vi "MPU panel.vi"() -> (0 "Error Out":errorcluster, 3 "VISA resource out":refnum<visa-resource-name>)   [LabVIEW 2016]
uses:
  <vilib>/Math Plots/3D Math Plots/3D Scatter/3D Scatter XCtrl/3D Scatter.xctl
  <vilib>/BLE/type_def/connection_status_bundle.ctl
  <vilib>/BLE/type_def/address_type.ctl
  Typedef/MPU panel - States.ctl
  Typedef/BLE char handle.ctl
  <vilib>/Math Plots/3D Math Plots/3D Scatter/3D Scatter Datatype/Public/Plot Helper (Vector).vi
  <vilib>/Math Plots/3D Math Plots/3D Scatter/3D Scatter Datatype/3D Scatter Datatype.lvclass
panel:
  in  "VISA resource in":refnum<visa-resource-name>
  in  "Calib Gyro":bool
  in  "Calib Mag":bool
  in  "Calib Accel":bool
  out "GyroZ":dbl caption="Z" format="%#_gdps"
  out "GyroY":dbl caption="Y" format="%#_gdps"
  out "GyroX":dbl caption="X" format="%#_gdps"
  out "Gyroscope Chart":cluster{"[0]":dbl, "[1]":dbl, "[2]":dbl}(graph)
  out "AccZ":dbl caption="Z" format="%#_gg"
  out "AccY":dbl caption="Y" format="%#_gg"
  out "AccX":dbl caption="X" format="%#_gg"
  out "Accelerometer Chart":cluster{"[0]":dbl, "[1]":dbl, "[2]":dbl}(graph)
  in  "Connection Status":T1={"MAC Address"="", "cnx handle"=0, "cnx flags"=0, "Address Type"=125, "Connection Interval (ms)"=125, "Timeout(ms)"=125, "Latency"=0, "bonding handle"=0} {"Address Type" items=["Public", "Random"]}
  in  "Clear Plot":bool
  out "3D Mag Scatter":refnum<class "3D Plot Datatype.lvclass">[](xcontrol)
  in  "Acquire MPU":bool
  # "Points [N]"
  # "Points [N]"
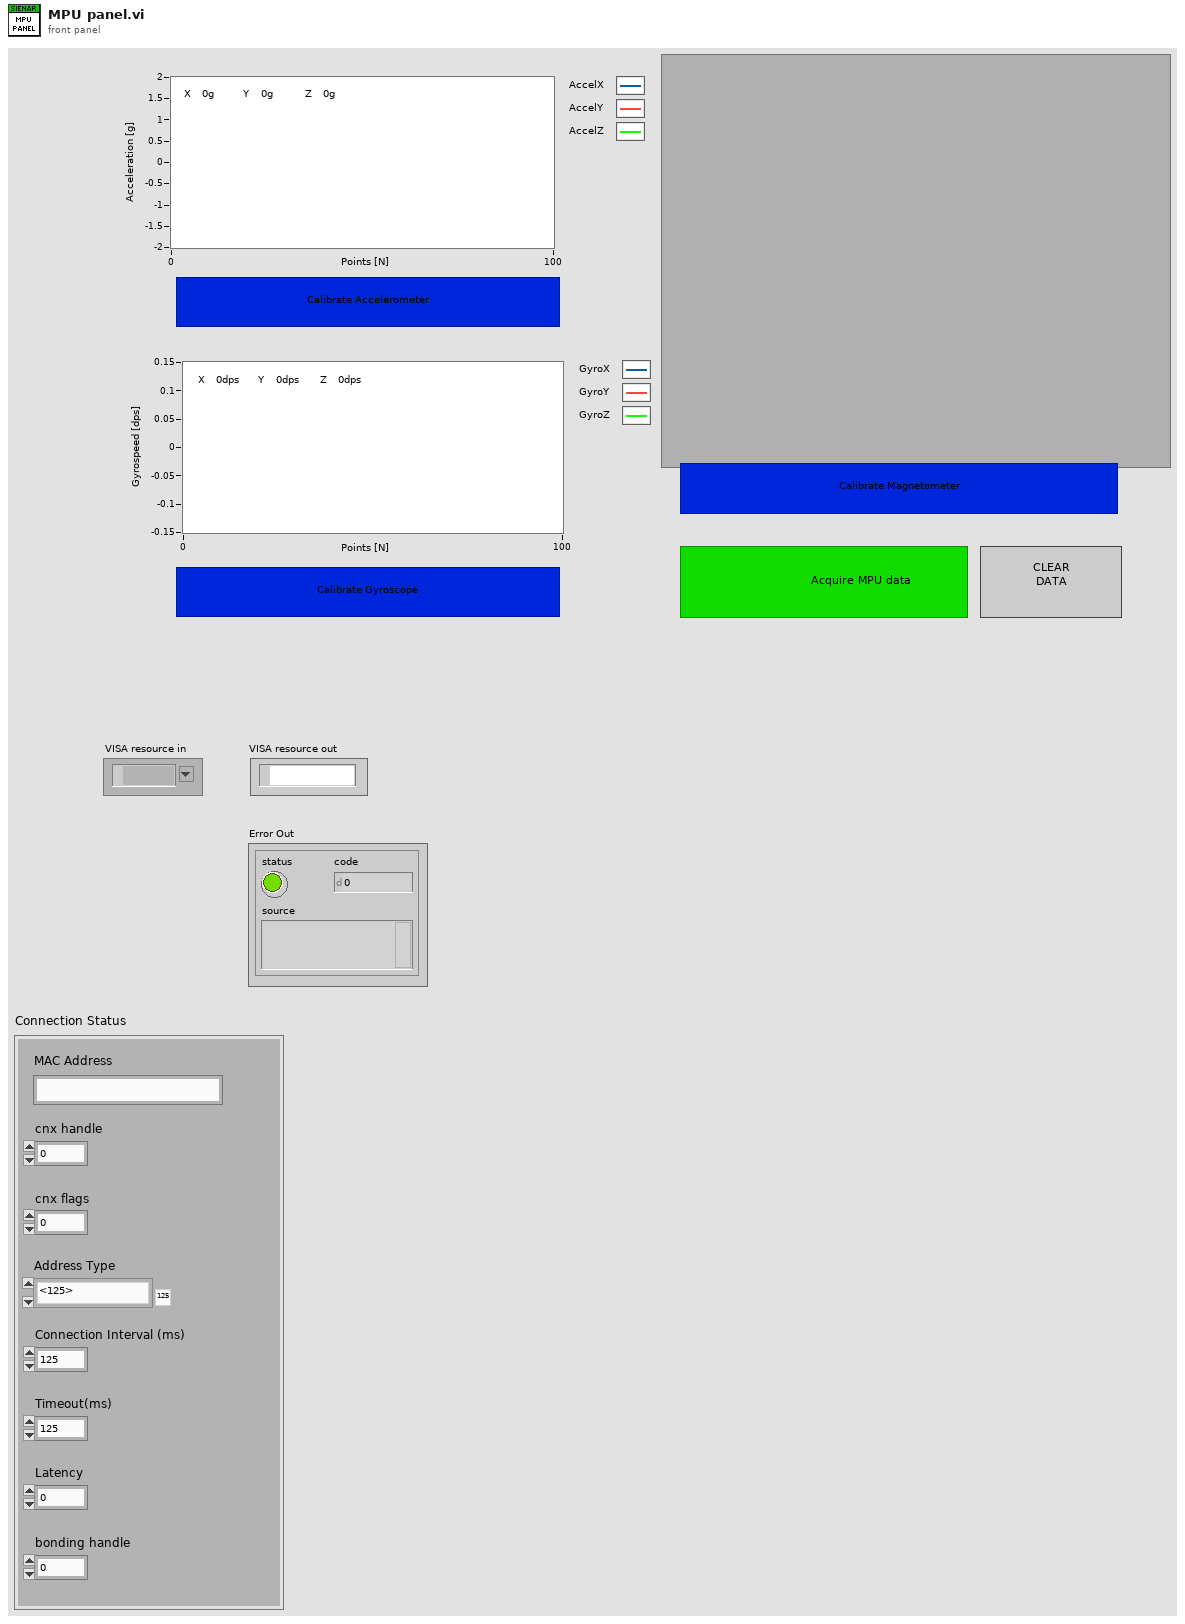
[diagram p1: front panel]
types:
  T1 = typedef "connection_status_bundle.ctl" = cluster{"MAC Address":string, "cnx handle":u8, "cnx flags":u8, "Address Type":T2, "Connection Interval (ms)":u16, "Timeout(ms)":u16, "Latency":u16, "bonding handle":u8}
  T2 = typedef "address_type.ctl" = u8
  T3 = typedef "MPU panel - States.ctl" = enum16{"Read MPU data", "Stop", "Calib Accelerometer", "Calib Gyroscope", "Calib Magnetometer", "Clear Plots", "Exit"}
  T4 = typedef "BLE char handle.ctl" = u16
  T5 = cluster{"AccelData":cluster{"AccelX":i16, "AccelY":i16, "AccelZ":i16}, "GyroData":cluster{"GyroX":i16, "GyroY":i16, "GyroZ":i16}, "MagData":cluster{"MagX":i16, "MagY":i16, "MagZ":i16}}
  T6 = cluster{"AccelData":cluster{"AccelX":dbl, "AccelY":dbl, "AccelZ":dbl}, "GyroData":cluster{"GyroX":dbl, "GyroY":dbl, "GyroZ":dbl}, "MagData":cluster{"MagX":dbl, "MagY":dbl, "MagZ":dbl}}
  T7 = cluster{"AccelX":dbl, "AccelY":dbl, "AccelZ":dbl}
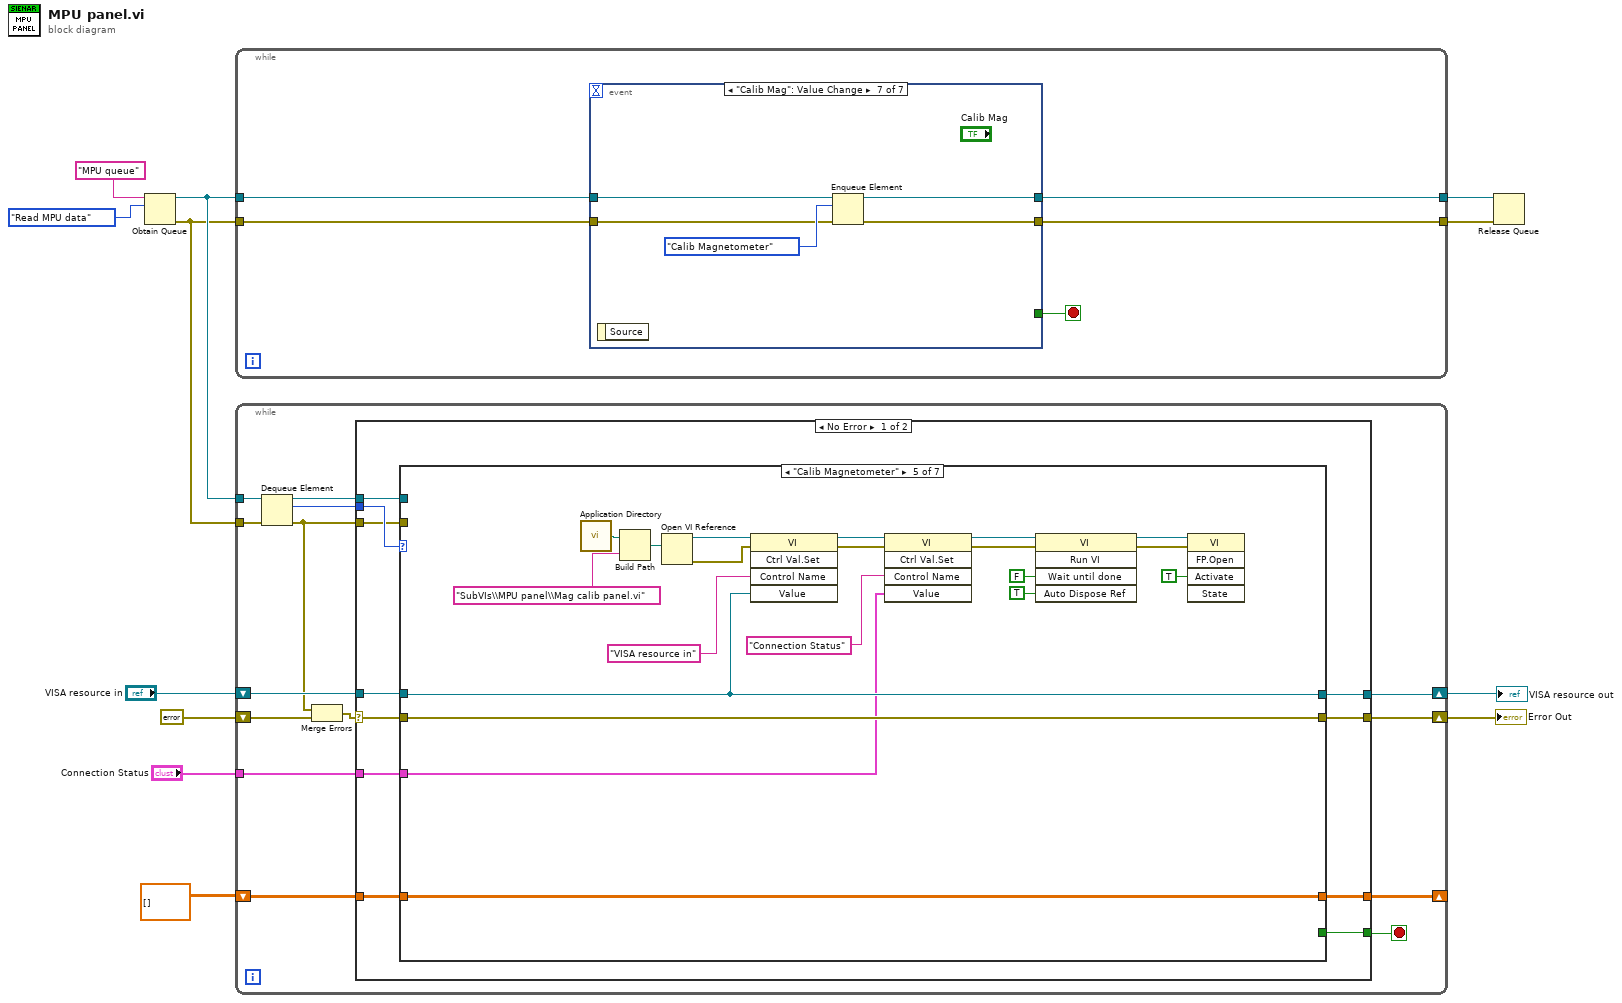
[diagram p0: block diagram]
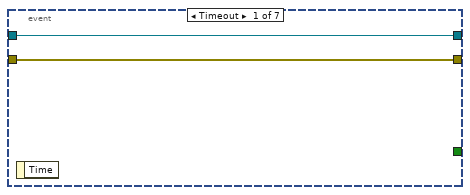
[diagram p2: hidden frame]
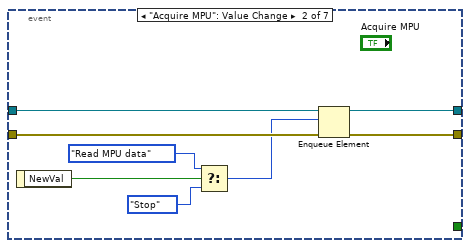
[diagram p3: hidden frame]
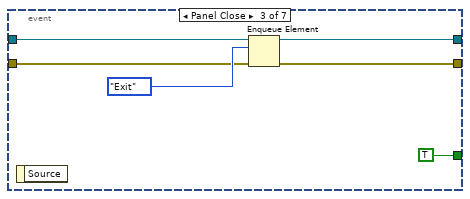
[diagram p4: hidden frame]
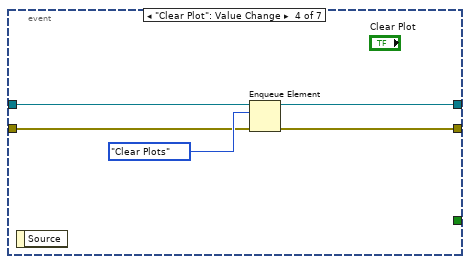
[diagram p5: hidden frame]
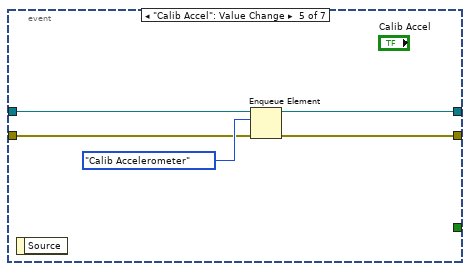
[diagram p6: hidden frame]
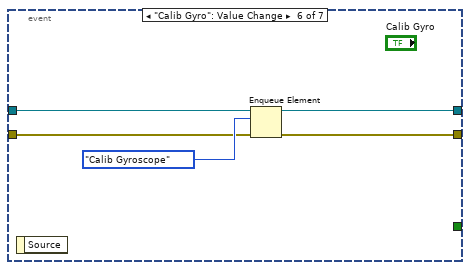
[diagram p7: hidden frame]
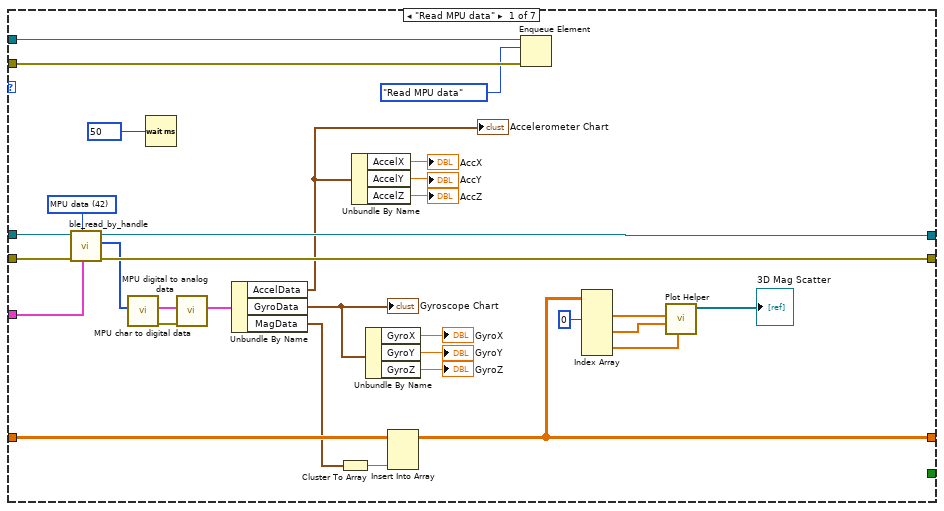
[diagram p8: hidden frame]
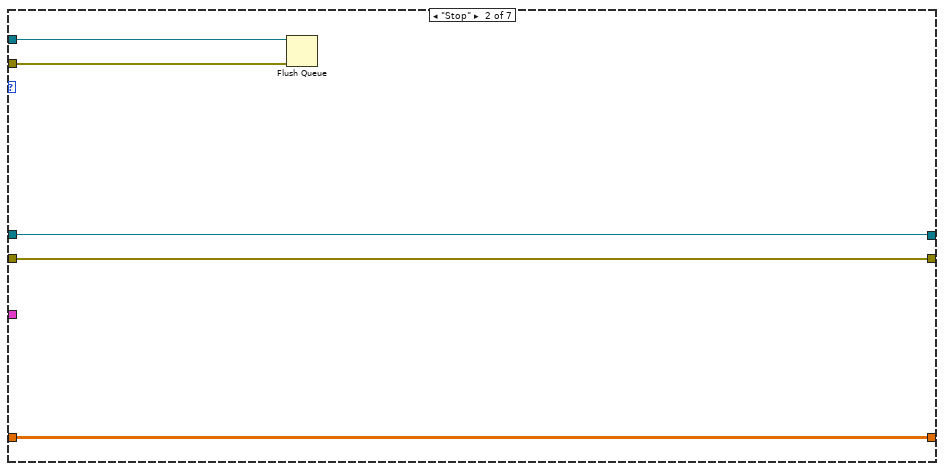
[diagram p9: hidden frame]
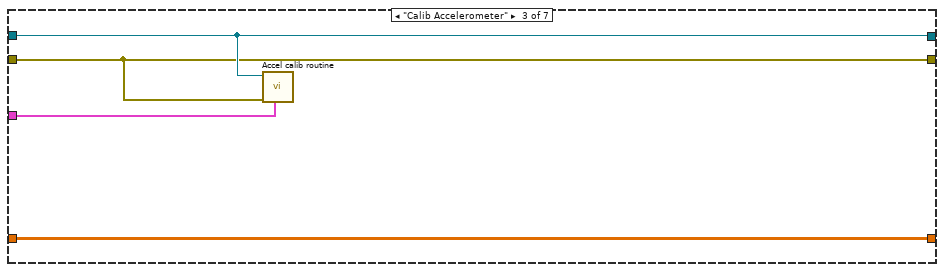
[diagram p10: hidden frame]
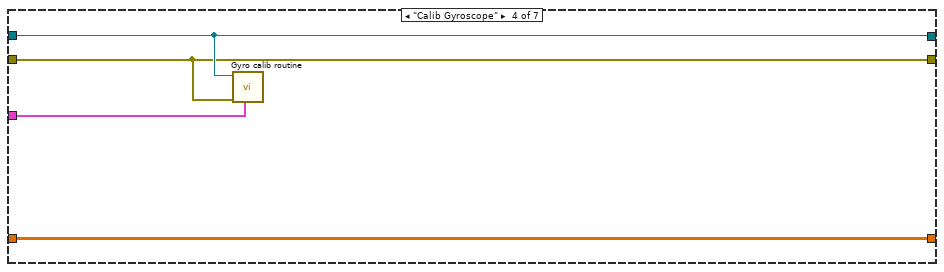
[diagram p11: hidden frame]
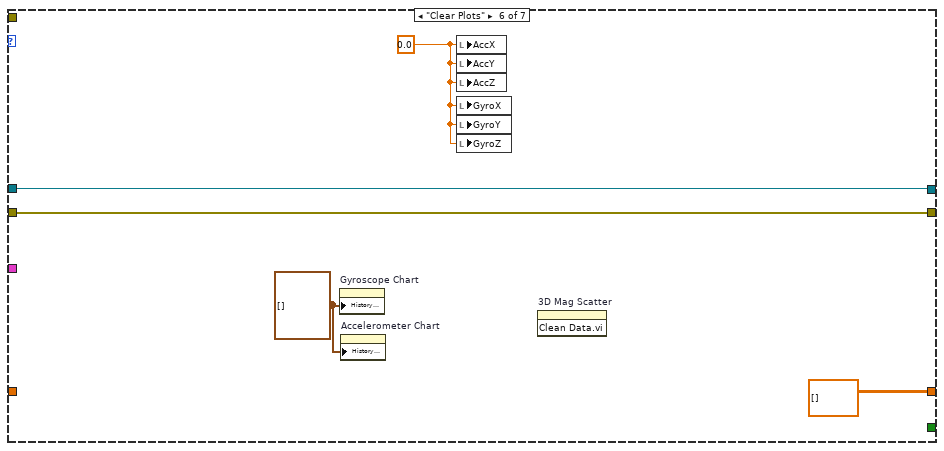
[diagram p12: hidden frame]
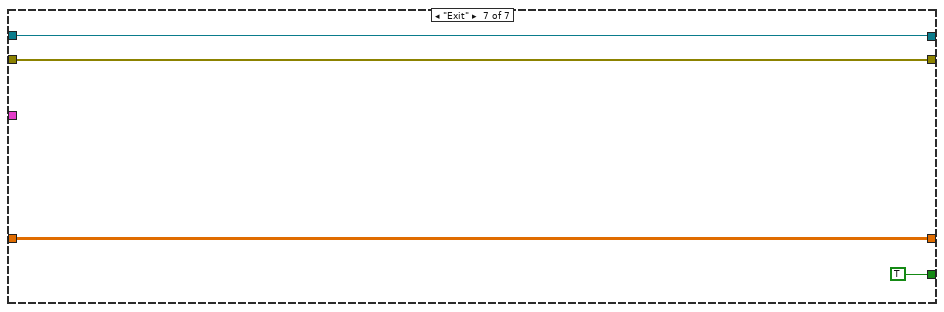
[diagram p13: hidden frame]
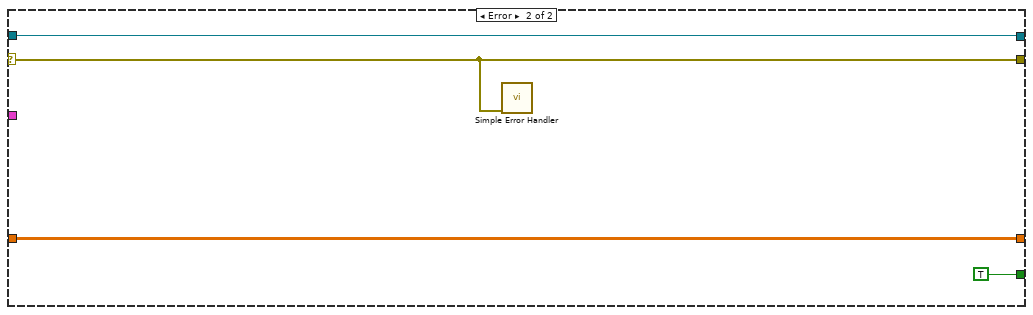
[diagram p14: hidden frame]
diagram:
  n1 = Obtain Queue(name (unnamed)="MPU queue", element data type=MPU_panel_-_States."Read MPU data") -> (queue out=w9:refnum<queue>, error out=w8:errorcluster)  [unwired: 3 in, 1 out]
  n2 = while {
    tunnel: w9 -> [w17]
    tunnel: w8 -> [w16]
    tunnel: [w15] -> w11
    tunnel: [w14] -> w10
    stop <- w13 stop-if-true
    n3 = event shown="[6] \"Calib Mag\": Value Change" {
      selector: _ -> [_ _ _ _ _ _ _]
      dyn-events: _ -> [_ _ _ _ _ _ _]
      timeout: _ -> [_ _ _ _ _ _ _]
      tunnel: w17 -> [w19 w27 w31 w37 w42 w47 w52]
      tunnel: w16 -> [w18 w26 w30 w36 w41 w46 w51]
      tunnel: [w18 w25 w29 w35 w40 w45 w50] -> w14
      tunnel: [w19 w24 w28 w34 w39 w44 w49] -> w15
      tunnel: [_ _ TRUE _ _ _ _] -> w13
      event Timeout {
        n4 = event-data() -> ()  [unwired: 1 in, 1 out]
      }
      event "Acquire MPU": Value Change {
        n5 = event-data() -> ("NewVal"=w23:bool)  [unwired: 1 in]
        n6 = Select(t=MPU_panel_-_States."Read MPU data", s=w23, f=MPU_panel_-_States."Stop") -> (s? t:f=w20:T3)
        n7 = Enqueue Element(queue=w27, element=w20, error in (no error)=w26) -> (queue out=w24:refnum<queue>, error out=w25:errorcluster)  [unwired: 1 in, 1 out]
      }
      event Panel Close {
        n8 = event-data() -> ()  [unwired: 1 in, 1 out]
        n9 = Enqueue Element(queue=w31, element=MPU_panel_-_States."Exit", error in (no error)=w30) -> (queue out=w28:refnum<queue>, error out=w29:errorcluster)  [unwired: 1 in, 1 out]
      }
      event "Clear Plot": Value Change {
        n10 = event-data() -> ()  [unwired: 1 in, 1 out]
        n11 = Enqueue Element(queue=w37, element=MPU_panel_-_States."Clear Plots", error in (no error)=w36) -> (queue out=w34:refnum<queue>, error out=w35:errorcluster)  [unwired: 1 in, 1 out]
      }
      event "Calib Accel": Value Change {
        n12 = event-data() -> ()  [unwired: 1 in, 1 out]
        n13 = Enqueue Element(queue=w42, element=MPU_panel_-_States."Calib Accelerometer", error in (no error)=w41) -> (queue out=w39:refnum<queue>, error out=w40:errorcluster)  [unwired: 1 in, 1 out]
      }
      event "Calib Gyro": Value Change {
        n14 = event-data() -> ()  [unwired: 1 in, 1 out]
        n15 = Enqueue Element(queue=w47, element=MPU_panel_-_States."Calib Gyroscope", error in (no error)=w46) -> (queue out=w44:refnum<queue>, error out=w45:errorcluster)  [unwired: 1 in, 1 out]
      }
      event "Calib Mag": Value Change {
        n16 = event-data() -> ()  [unwired: 1 in, 1 out]
        n17 = Enqueue Element(queue=w52, element=MPU_panel_-_States."Calib Magnetometer", error in (no error)=w51) -> (queue out=w49:refnum<queue>, error out=w50:errorcluster)  [unwired: 1 in, 1 out]
      }
    }
  }
  n18 = while {
    tunnel: w9 -> [w67]
    tunnel: w8 -> [w66]
    shift-right: [w62] -> w4
    shift-left: "VISA resource in" -> [w63]
    shift-right: [w61] -> w5
    shift-left: errorcluster {"status"=FALSE, "code"=0, "source"=""} ("Error In") -> [w56]
    tunnel: "Connection Status" -> [w59]
    shift-right: [w58] -> _
    shift-left: dbl[][] [] -> [w57]
    stop <- w64 stop-if-true
    n19 = Dequeue Element(queue=w67, error in (no error)=w66) -> (queue out=w60:refnum<queue>, element=w65:T3, error out=w54:errorcluster)  [unwired: 1 in, 1 out]
    n20 = Merge Errors(w54, w56) -> (w55:errorcluster)
    n21 = case shown="No Error" w55 {
      selector: w55 -> [w68 w152]
      tunnel: w65 -> [w78 _]
      tunnel: [w77 TRUE] -> w64
      tunnel: w63 -> [w76 w155]
      tunnel: [w75 w155] -> w62
      tunnel: [w74 w152] -> w61
      tunnel: w54 -> [w73 _]
      tunnel: w60 -> [w72 _]
      tunnel: w59 -> [w71 _]
      tunnel: [w70 w154] -> w58
      tunnel: w57 -> [w69 w154]
      frame No Error {
        n22 = case shown="\"Calib Magnetometer\"" w78 {
          tunnel: [_ _ _ _ _ _ TRUE] -> w77
          tunnel: w76 -> [w109 w112 w116 w121 w137 w147 w150]
          tunnel: w68 -> [w108 w111 w115 w119 w142 w146 w149]
          tunnel: [w107 w112 w116 w121 w137 w147 w150] -> w75
          tunnel: [w106 w111 w115 w119 w142 w146 w149] -> w74
          tunnel: w73 -> [w104 w113 _ _ _ _ _]
          tunnel: w72 -> [w105 w114 _ _ _ _ _]
          tunnel: w71 -> [w100 _ w118 w120 w133 _ _]
          tunnel: [w98 w110 w117 w122 w132 dbl[][] [] w148] -> w70
          tunnel: w69 -> [w99 w110 w117 w122 w132 _ w148]
          frame "Read MPU data" {
            w79 = T4 42 items=["MPU data"=42, "MPU data - DESCR"=43, "Accel calib parameters"=45, "Gyro calib parameters"=47, "Mag calib parameters - 1"=49, "Mag calib parameters - 2"=51, "YPR"=53, "YPR - DESCR"=54, "Strain sensors"=56, "Strain sensors - DESCR"=57, "Wristband"=59, "Wristband - DESCR"=60] ("BLE char handle")
            n23 = call <vilib>:"ble_read_by_handle.vi"("Connection Status"=w100, "Handle"=w79, "error in (no error)"=w108, "COM Bluegiga in"=w109) -> ("error out"=w106:errorcluster, "characteristic value"=w80:u8[], "COM Bluegiga out"=w107:refnum<visa-resource-name>)  [unwired: 5 in]
            n24 = call "MPU char to digital data.vi"("MPU characteristic data"=w80) -> ("Error Out"=w89:errorcluster, "Digital MPU data"=w90:T5)  [unwired: 9 in]
            n25 = Wait (ms)(milliseconds to wait=u32 50 ("Acquisition interval")) -> ()  [unwired: 1 out]
            n26 = call "MPU digital to analog data.vi"("Error In"=w89, "Digital MPU data"=w90) -> ("Analog MPU data"=w88:T6)  [unwired: 8 in, 1 out]
            n27 = Unbundle By Name(w88) -> ("AccelData"=w87:T7, "GyroData"=w83:cluster{"GyroX":dbl, "GyroY":dbl, "GyroZ":dbl}, "MagData"=w82:cluster{"MagX":dbl, "MagY":dbl, "MagZ":dbl})
            "Accelerometer Chart" <- w87
            "Gyroscope Chart" <- w83
            n28 = Cluster To Array(cluster=w82) -> (array=w81:dbl[])
            n29 = Unbundle By Name(w87) -> ("AccelX"=→"AccX":dbl, "AccelY"=→"AccY":dbl, "AccelZ"=→"AccZ":dbl)
            n30 = Unbundle By Name(w83) -> ("GyroX"=→"GyroX":dbl, "GyroY"=→"GyroY":dbl, "GyroZ"=→"GyroZ":dbl)
            n31 = Insert Into Array(array=w99, new element=w81) -> (w98:dbl[][])  [unwired: 2 in]
            n32 = Enqueue Element(queue=w105, element=MPU_panel_-_States."Read MPU data", error in (no error)=w104) -> ()  [unwired: 1 in, 3 out]
            n33 = Index Array(array=w98, index (col) #1=0 ("disabled index (col)")) -> (element #1=w96:dbl[], element #2=w95:dbl[], element #3=w94:dbl[])  [unwired: 5 in]
            n34 = call-poly <vilib>:"Plot Helper.vi"("z vector"=w94, "y vector"=w95, "x vector"=w96) -> ("3D Plot lvclass Array out"=→"3D Mag Scatter":refnum<class "3D Plot Datatype.lvclass">[])  [unwired: 3 in, 5 out]
          }
          frame "Stop" {
            n35 = Flush Queue(queue=w114, error in (no error)=w113) -> ()  [unwired: 3 out]
          }
          frame "Calib Accelerometer" {
            n36 = call "Accel calib routine.vi"("Connection Status"=w118, "Error In"=w115, "VISA resource in"=w116) -> ()  [unwired: 9 in]
          }
          frame "Calib Gyroscope" {
            n37 = call "Gyro calib routine.vi"("Connection Status"=w120, "Error In"=w119, "VISA resource in"=w121) -> ()  [unwired: 9 in]
          }
          frame "Calib Magnetometer" {
            n38 = call <vilib>:"Application Directory.vi"() -> ("Application Directory"=w141:path)
            n39 = Build Path(base path=w141, name or relative path="SubVIs\\MPU panel\\Mag calib panel.vi") -> (appended path=w140:path)
            n40 = Open VI Reference(vi path=w140) -> (vi reference=w131:refnum<vi>, error out=w130:errorcluster)  [unwired: 5 in]
            n41 = invoke class="VI" method="Ctrl Val.Set"(reference=w131, error in=w130, "Control Name"="VISA resource in", "Value"=w137) -> (reference out=w135:refnum<vi>, error out=w136:errorcluster)  [unwired: 1 in, 3 out]
            n42 = invoke class="VI" method="Ctrl Val.Set"(reference=w135, error in=w136, "Control Name"="Connection Status", "Value"=w133) -> (reference out=w124:refnum<vi>, error out=w123:errorcluster)  [unwired: 1 in, 3 out]
            n43 = invoke class="VI" method="Run VI"(reference=w124, error in=w123, "Wait until done"=FALSE ("Wait Until Done"), "Auto Dispose Ref"=TRUE ("Auto Dispose Reference")) -> (reference out=w127:refnum<vi>, error out=w126:errorcluster)  [unwired: 1 in, 3 out]
            n44 = invoke class="VI" method="FP.Open"(reference=w127, error in=w126, "Activate"=TRUE ("Activate?")) -> ()  [unwired: 2 in, 5 out]
          }
          frame "Clear Plots" {
            w143 = 0.0
            w144 = cluster{"[0]":dbl, "[1]":dbl, "[2]":dbl}[] [] ("History Data")
            n45 = property on="Gyroscope Chart" class="WFChart (strict)"("History Data"=w144) -> ()  [unwired: 2 in, 2 out]
            n46 = property on="Accelerometer Chart" class="WFChart (strict)"("History Data"=w144) -> ()  [unwired: 2 in, 2 out]
            n47 = local write "AccX"(w143) -> ()
            n48 = local write "AccY"(w143) -> ()
            n49 = local write "AccZ"(w143) -> ()
            n50 = local write "GyroX"(w143) -> ()
            n51 = local write "GyroY"(w143) -> ()
            n52 = local write "GyroZ"(w143) -> ()
            n53 = invoke on="3D Mag Scatter" class="3D Scatter (strict)" method="Clean Data.vi"() -> ()  [unwired: 3 in, 3 out]
          }
          frame "Exit" {
          }
        }
      }
      frame Error {
        n54 = call <vilib>:"Simple Error Handler.vi"("error in (no error)"=w152) -> ()  [unwired: 4 in, 5 out]
      }
    }
  }
  "Error Out" <- w5
  "VISA resource out" <- w4
  n55 = Release Queue(queue=w11, error in (no error)=w10) -> ()  [unwired: 1 in, 3 out]
